vi "stateUpdated.vi"(8 "error in (no error)":errorcluster, 11 "StaticOutputEditor in":refnum<class "StaticOutputEditor.lvclass">) -> (0 "error out":errorcluster, 3 "StaticOutputEditor out":refnum<class "StaticOutputEditor.lvclass">)   [LabVIEW 2011, in "Views.lvlib" / "ScriptEditor.lvlib" / "StaticOutputEditor.lvclass"]
uses:
  StaticOutputEditor.lvclass
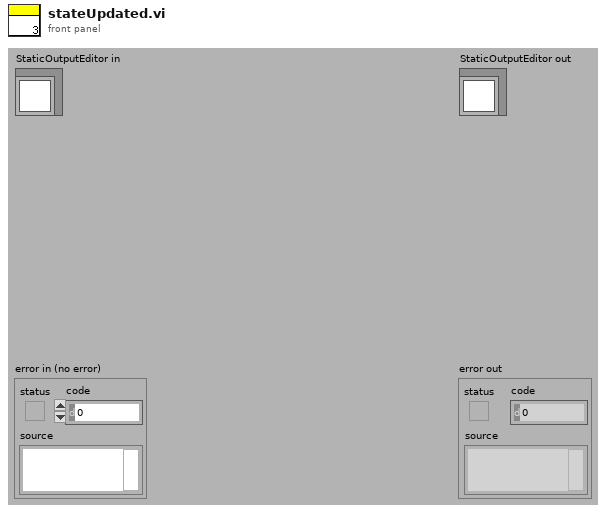
[diagram p1: front panel]
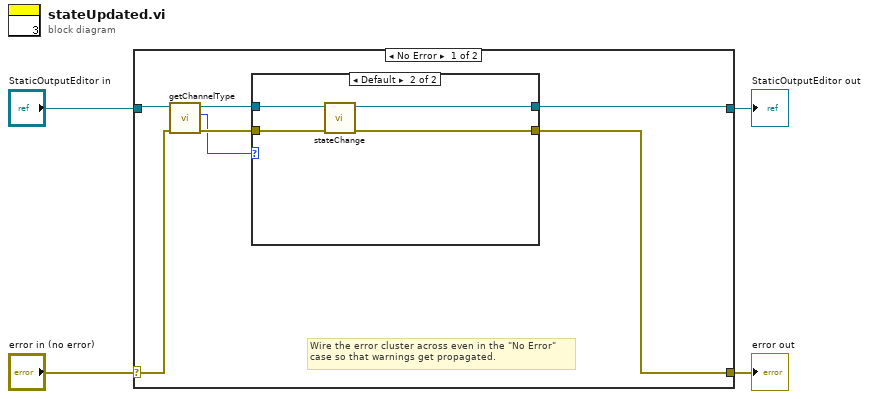
[diagram p0: block diagram]
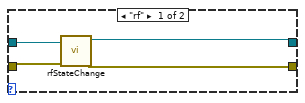
[diagram p2: hidden frame]
diagram:
  n1 = case shown="No Error" "error in (no error)" {
    selector: "error in (no error)" -> [w6 w21]
    tunnel: [w7 w21] -> w3
    tunnel: [w9 w20] -> w1
    tunnel: "StaticOutputEditor in" -> [w11 w20]
    frame No Error {
      # "Wire the error cluster across even in the \"No Error\"\ncase so that warnings get propagated."
      n2 = call "getChannelType.vi"("error in (no error)"=w6, "StaticOutputEditor in"=w11) -> ("error out"=w8:errorcluster, "channel_type"=w5:enum16{"ao", "do", "ai", "di", "rf"}, "StaticOutputEditor out"=w10:refnum<class "StaticOutputEditor.lvclass">)  [unwired: 7 in]
      n3 = case shown="Default" w5 {
        tunnel: w10 -> [w15 w19]
        tunnel: [w14 w18] -> w9
        tunnel: w8 -> [w12 w17]
        tunnel: [w13 w16] -> w7
        frame "rf" {
          n4 = call "rfStateChange.vi"("error in (no error)"=w12, "StaticOutputEditor in"=w15) -> ("error out"=w13:errorcluster, "StaticOutputEditor out"=w14:refnum<class "StaticOutputEditor.lvclass">)  [unwired: 8 in]
        }
        frame Default {
          n5 = call "stateChange.vi"("error in (no error)"=w17, "StaticOutputEditor in"=w19) -> ("error out"=w16:errorcluster, "StaticOutputEditor out"=w18:refnum<class "StaticOutputEditor.lvclass">)  [unwired: 8 in]
        }
      }
    }
    frame Error {
    }
  }
  "error out" <- w3
  "StaticOutputEditor out" <- w1
